vi "Send Command.vi"(5 "Message":string, 7 "Command":T1=enum."Start Run") -> (1 "Error":string, 3 "Data":string)   [LabVIEW 2012]
uses:
  Type/_Server Command.ctl
  Type/_Server Control Type.ctl
panel:
  out "Run Time (ms)":u32
  # "A DLL function to send a command to the Server"
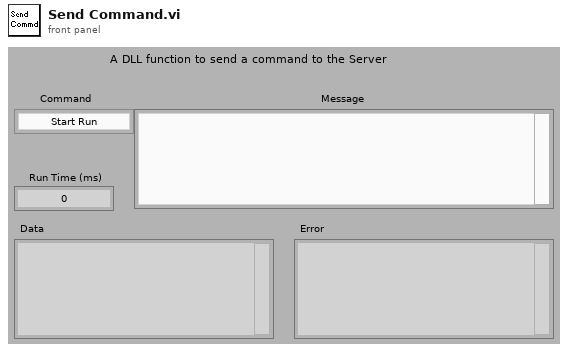
[diagram p1: front panel]
types:
  T1 = typedef "_Server Command.ctl" = enum16{"Hide Server", "Show Server", "Close Server", "Start Run", "Stop Run", "Runtime Update", "Get Data", "Get Status", "Get Table", "Set Table", "Get Configuration", "Reserved", "Get Memory Map", "Read ADC", "Set Oscillator", "Reboot", "Backup Firmware", "Update Firmware", "Auxiliary Update", "System Status", "Start System", "Shutdown System", "Start LC Equilibration", "Get LC Status", "Get LC Configuration", "Get LC Method Contents", "Rinse Autosampler", "Pump OnOff", "Oven OnOff", "Get LC Error", "Clear LC Error", "Lock Server", "Get Current Method", "Get Real Time Data", "Connect LC", "Disconnect LC"}
  T2 = typedef "_Server Control Type.ctl" = enum16{"Command", "Boolean", "Text"}
  T3 = typedef "_Server Reference.ctl" = cluster{"Server Reference":refnum<vi>, "Command Ref":refnum<vi>, "Message Ref":refnum<vi>, "Ready Ref":refnum<vi>, "Locked Ref":refnum<vi>, "Data Ref":refnum<vi>, "Error Ref":refnum<vi>, "Busy Ref":refnum<vi>}
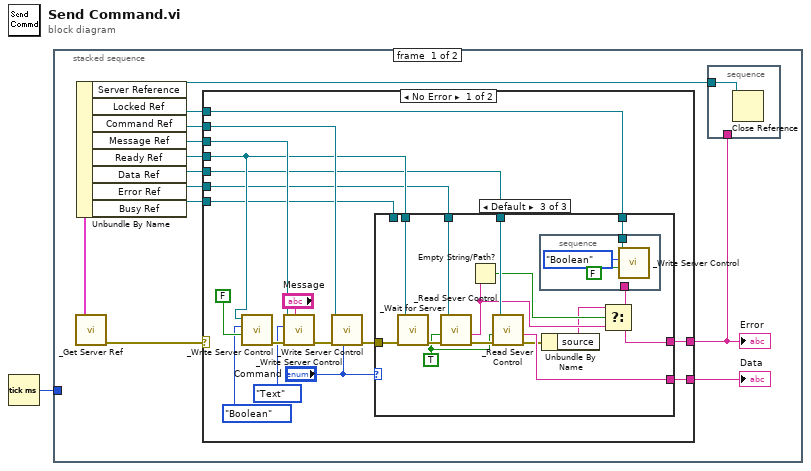
[diagram p0: block diagram]
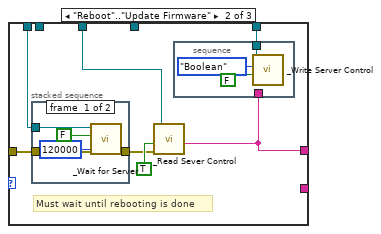
[diagram p3: hidden frame]
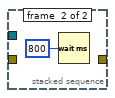
[diagram p4: hidden frame]
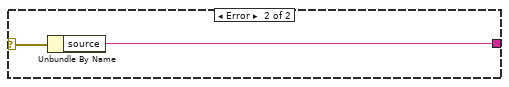
[diagram p5: hidden frame]
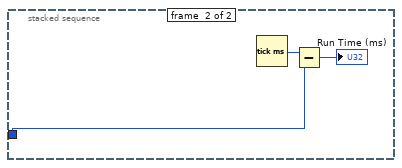
[diagram p6: hidden frame]
diagram:
  n1 = Tick Count (ms)() -> (millisecond timer value=w1:u32)
  n2 = stacked-sequence {
    tunnel: w1 -> [_ w67]
    frame #0 {
      n3 = call "_Get Server Ref.vi"() -> ("error out"=w3:errorcluster, "Server Ref"=w8:T3)  [unwired: 1 in, 5 out]
      n4 = Unbundle By Name(w8) -> ("Server Reference"=w6:refnum<vi>, "Locked Ref"=w7:refnum<vi>, "Command Ref"=w9:refnum<vi>, "Message Ref"=w10:refnum<vi>, "Ready Ref"=w11:refnum<vi>, "Data Ref"=w12:refnum<vi>, "Error Ref"=w13:refnum<vi>, "Busy Ref"=w4:refnum<vi>)
      n5 = case shown="No Error" w3 {
        selector: w3 -> [_ w66]
        tunnel: [w16 w65] -> w2
        tunnel: [w27 _] -> w5
        tunnel: w9 -> [w25 _]
        tunnel: w10 -> [w26 _]
        tunnel: w11 -> [w24 _]
        tunnel: w12 -> [w20 _]
        tunnel: w13 -> [w21 _]
        tunnel: w7 -> [w15 _]
        tunnel: w4 -> [w17 _]
        frame No Error {
          n6 = call "_Write Server Control.vi"("Boolean (F)"=FALSE, "Control Type"=_Server_Control_Type."Boolean", "Control Ref"=w24) -> ("error out"=w30:errorcluster)  [unwired: 4 in, 2 out]
          n7 = call "_Write Server Control.vi"("Text"="Message", "error in (no error)"=w30, "Control Type"=_Server_Control_Type."Text", "Control Ref"=w26) -> ("error out"=w29:errorcluster)  [unwired: 2 in, 3 out]
          n8 = call "_Write Server Control.vi"("Command"="Command", "error in (no error)"=w29, "Control Ref"=w25) -> ("error out"=w28:errorcluster)  [unwired: 3 in, 3 out]
          n9 = case shown="Default" "Command" {
            tunnel: w28 -> [_ w38 w61]
            tunnel: [_ _ w54] -> w27
            tunnel: w24 -> [_ _ w59]
            tunnel: w21 -> [_ w34 w58]
            tunnel: w20 -> [_ _ w55]
            tunnel: [_ w32 w48] -> w16
            tunnel: w17 -> [_ w37 _]
            tunnel: w15 -> [_ w33 w53]
            frame "Close Server" {
            }
            frame "Reboot".."Update Firmware" {
              # "Must wait until rebooting is done"
              n10 = stacked-sequence {
                tunnel: w38 -> [w46 _]
                tunnel: w37 -> [w45 _]
                tunnel: [w42 _] -> w35
                frame #0 {
                  n11 = call "_Wait for Server.vi"("error in"=w46, "Timeout (8s)"=u32 120000 ("Timeout (5s)"), "For Ready Signal? (T)"=FALSE, "Indicator Ref"=w45) -> ("error out"=w42:errorcluster)  [unwired: 3 out]
                }
                frame #1 {
                  n12 = Wait (ms)(milliseconds to wait=u32 800) -> ()  [unwired: 1 out]
                }
              }
              n13 = call "_Read Sever Control.vi"("error in (no error)"=w35, "Text? (F)"=TRUE, "Control Ref"=w34) -> ("Text"=w32:string)  [unwired: 1 in, 3 out]
              n14 = stacked-sequence {
                tunnel: w33 -> [w41]
                tunnel: w32 -> [_]
                frame #0 {
                  n15 = call "_Write Server Control.vi"("Boolean (F)"=FALSE, "Control Type"=_Server_Control_Type."Boolean", "Control Ref"=w41) -> ()  [unwired: 4 in, 3 out]
                }
              }
            }
            frame Default {
              w56 = TRUE
              n16 = call "_Wait for Server.vi"("error in"=w61, "Indicator Ref"=w59) -> ("error out"=w60:errorcluster)  [unwired: 2 in, 3 out]
              n17 = call "_Read Sever Control.vi"("error in (no error)"=w60, "Text? (F)"=w56, "Control Ref"=w58) -> ("error out"=w57:errorcluster, "Text"=w51:string)  [unwired: 1 in, 2 out]
              n18 = Empty String/Path?(string/path=w51) -> (empty?=w52:bool)
              n19 = call "_Read Sever Control.vi"("error in (no error)"=w57, "Text? (F)"=w56, "Control Ref"=w55) -> ("error out"=w50:errorcluster, "Text"=w54:string)  [unwired: 1 in, 2 out]
              n20 = Unbundle By Name(w50) -> ("source"=w49:string)
              n21 = Select(t=w49, s=w52, f=w51) -> (s? t:f=w48:string)
              n22 = stacked-sequence {
                tunnel: w53 -> [w64]
                tunnel: w48 -> [_]
                frame #0 {
                  n23 = call "_Write Server Control.vi"("Boolean (F)"=FALSE, "Control Type"=_Server_Control_Type."Boolean", "Control Ref"=w64) -> ()  [unwired: 4 in, 3 out]
                }
              }
            }
          }
        }
        frame Error {
          n24 = Unbundle By Name(w66) -> ("source"=w65:string)
        }
      }
      "Error" <- w2
      "Data" <- w5
      n25 = stacked-sequence {
        tunnel: w6 -> [w14]
        tunnel: w2 -> [_]
        frame #0 {
          n26 = Close Reference(reference=w14) -> ()  [unwired: 1 in, 1 out]
        }
      }
    }
    frame #1 {
      n27 = Tick Count (ms)() -> (millisecond timer value=w69:u32)
      n28 = Subtract(x=w69, y=w67) -> (x-y=→"Run Time (ms)":u32)
    }
  }
